vi "USB2XXX_LINEX_MasterSimpleWriteReadTest.vi"() -> ()   [LabVIEW 2010]
panel:
  out "Readed Data Num":i32
  out "Read Data(Hex)":string
  in  "Read Data ID":u8=2
  in  "Write Data(Hex)":string="11 22 33 44 55 66 77 88"
  in  "CheckType":u8
  in  "Write Data ID":u8=1
  in  "BaudRate":u32=19200
  in  "Channel Index":u8(ring) items=["LIN1", "LIN2"]
  in  "Device Index":i32(ring) items=["0", "1", "2", "3", "4", "5"]
  # "波特率一定要设置，否则程序可能出错"
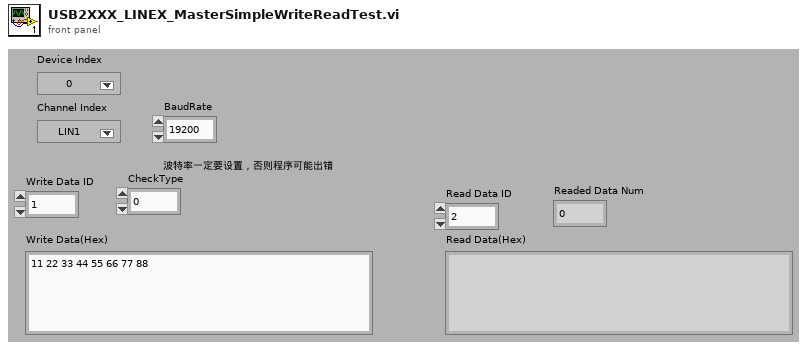
[diagram p1: front panel]
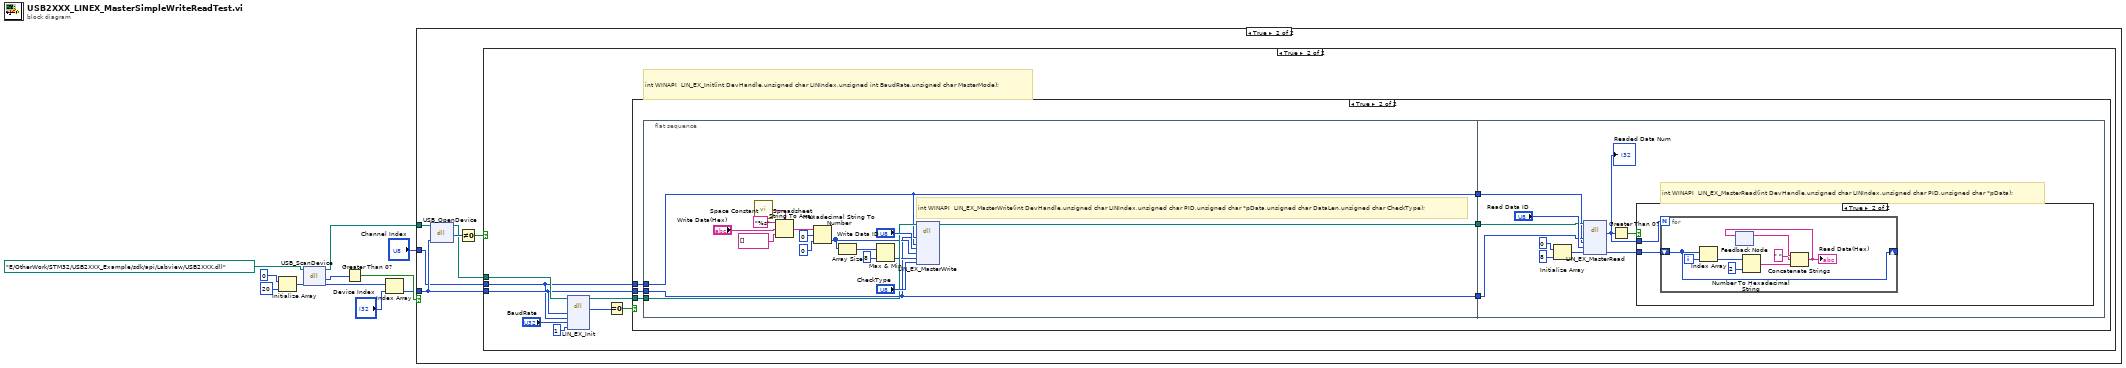
[diagram p0: block diagram]
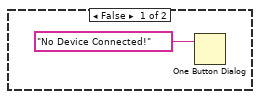
[diagram p2: hidden frame]
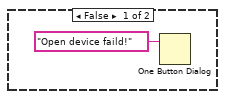
[diagram p3: hidden frame]
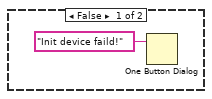
[diagram p4: hidden frame]
diagram:
  n1 = Initialize Array(0, 20 ("dimension size")) -> (w9:i32[])
  n2 = dll-call lib="E:/OtherWork/STM32/USB2XXX_Example/examples/Labview/PublicFiles/USB2XXX.dll" fn="USB_ScanDevice"(path in=path "E:/OtherWork/STM32/USB2XXX_Example/sdk/api/Labview/USB2XXX.dll", "pDevNum"=w9) -> (path out=w3:path, "return type"=w7:i32, "pDevNum"=w6:i32[])  [unwired: 2 in, 1 out]
  n3 = Greater Than 0?(x=w7) -> (x > 0?=w4:bool)
  n4 = Index Array(array=w6, index="Device Index") -> (element=w2:i32)
  n5 = case shown="True" w4 {
    tunnel: w3 -> [_ w18]
    tunnel: w2 -> [_ w14]
    tunnel: "Channel Index" -> [_ w13]
    frame False {
      n6 = One Button Dialog(message="No Device Connected!") -> ()  [unwired: 1 in, 1 out]
    }
    frame True {
      n7 = dll-call lib="E:/OtherWork/STM32/USB2XXX_Example/examples/Labview/PublicFiles/USB2XXX.dll" fn="USB_OpenDevice"(path in=w18, "DevIndex"=w14) -> (path out=w15:path, "return type"=w17:u8)  [unwired: 3 in, 1 out]
      n8 = Not Equal To 0?(x=w17) -> (x != 0?=w16:bool)
      n9 = case shown="True" w16 {
        tunnel: w15 -> [_ w25]
        tunnel: w14 -> [_ w21]
        tunnel: w13 -> [_ w20]
        frame False {
          n10 = One Button Dialog(message="Open device faild!") -> ()  [unwired: 1 in, 1 out]
        }
        frame True {
          # "int WINAPI  LIN_EX_Init(int DevHandle,unsigned char LINIndex,unsigned int BaudRate,unsigned char MasterMode);"
          n11 = dll-call lib="E:/OtherWork/STM32/USB2XXX_Example/examples/Labview/PublicFiles/USB2XXX.dll" fn="LIN_EX_Init"(path in=w25, "DevHandle"=w21, "LINIndex"=w20, "BaudRate"="BaudRate", "MasterMode"=u8 1) -> (path out=w22:path, "return type"=w24:i32)  [unwired: 6 in, 1 out]
          n12 = Equal To 0?(x=w24) -> (x = 0?=w23:bool)
          n13 = case shown="True" w23 {
            tunnel: w22 -> [_ w34]
            tunnel: w21 -> [_ w33]
            tunnel: w20 -> [_ w32]
            frame False {
              n14 = One Button Dialog(message="Init device faild!") -> ()  [unwired: 1 in, 1 out]
            }
            frame True {
              n15 = flat-sequence {
                tunnel: w34 -> [w49]
                tunnel: w33 -> [w36]
                tunnel: w32 -> [w35]
                tunnel: [w37] -> w31
                tunnel: [w36] -> w30
                tunnel: [w35] -> w29
                tunnel: w31 -> [w60]
                tunnel: w30 -> [w59]
                tunnel: w29 -> [w58]
                frame #0 {
                  # "int WINAPI  LIN_EX_MasterWrite(int DevHandle,unsigned char LINIndex,unsigned char PID,unsigned char *pData,unsigned char DataLen,unsigned char CheckType);"
                  n16 = call <vilib>:"Space Constant.vi"() -> ("String"=w44:string)
                  n17 = Spreadsheet String To Array(delimiter (Tab)=w44, format string="%s", spreadsheet string="Write Data(Hex)", array type (2D Dbl)=string[] []) -> (array=w47:string[])
                  n18 = Hexadecimal String To Number(string=w47, offset=0, default (0uL)=u8 0 ("default (0 U32)")) -> (number=w41:u8[])  [unwired: 1 out]
                  n19 = Array Size(array=w41) -> (size(s)=w40:i32)
                  n20 = Max & Min(x=w40, y=8) -> (min(x,y)=w38:i32)  [unwired: 1 out]
                  n21 = dll-call lib="E:/OtherWork/STM32/USB2XXX_Example/sdk/api/Labview/USB2XXX.*" fn="LIN_EX_MasterWrite"(path in=w49, "DevHandle"=w36, "LINIndex"=w35, "PID"="Write Data ID", "pData"=w41, "DataLen"=w38, "CheckType"="CheckType") -> (path out=w37:path)  [unwired: 9 in, 1 out]
                }
                frame #1 {
                  # "int WINAPI  LIN_EX_MasterRead(int DevHandle,unsigned char LINIndex,unsigned char PID,unsigned char *pData);"
                  n22 = Initialize Array(u8 0 ("element"), 8 ("dimension size")) -> (w55:u8[])
                  n23 = dll-call lib="E:/OtherWork/STM32/USB2XXX_Example/sdk/api/Labview/USB2XXX.*" fn="LIN_EX_MasterRead"(path in=w60, "DevHandle"=w59, "LINIndex"=w58, "PID"="Read Data ID", "pData"=w55) -> ("return type"=w52:i32, "pData"=w54:u8[])  [unwired: 5 in, 2 out]
                  "Readed Data Num" <- w52
                  n24 = Greater Than 0?(x=w52) -> (x > 0?=w57:bool)
                  n25 = case shown="True" w57 {
                    tunnel: w52 -> [_ w63]
                    tunnel: w54 -> [_ w62]
                    frame False {
                    }
                    frame True {
                      n26 = for {
                        N: w63 -> [_]
                        shift-right: [w64] -> _
                        shift-left: w62 -> [w64]
                        i -> [w71]
                        n27 = Index Array(array=w64, index=w71) -> (element=w70:u8)
                        n28 = feedback #1() -> (w68:string)  [unwired: 1 in]
                        n29 = Number To Hexadecimal String(1:i16 2 ("width (-)"), 2:w70) -> (0:w66:string)
                        n30 = Concatenate Strings(w68, " " ("string"), w66) -> (w65:string)
                        "Read Data(Hex)" <- w65
                        n31 = feedback-in #1(w65) -> ()
                      }
                    }
                  }
                }
              }
            }
          }
        }
      }
    }
  }
